vi "UIMessage AX Callback.vi"(4 "Variant":variant, 5 "Event Data":cluster{"msg":refnum<k7>}, 6 "Control Ref":refnum<k7>, 7 "Event Common Data":T2) -> ()   [LabVIEW 2020, in "TSnax.lvlib" / "Engine.lvclass"]
uses:
  Engine.lvclass
  UIMsg.ctl
  Engine.lvclass/Engine.ctl
  UIMessage/UIMessage.lvclass
  TSnax.lvlib
panel:
  out "Code":T1
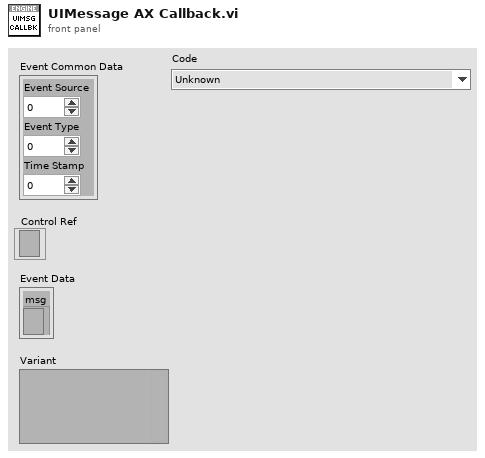
[diagram p1: front panel]
types:
  T1 = typedef "TSnax.lvlib/UIMsg.ctl" = enum16{"Unknown", "BreakOnUserRequest", "BreakOnBreakpoint", "BreakOnRunTimeError", "Trace", "TerminatingExecution", "AbortingExecution", "KillingExecutionThreads", "EndExecution", "ShutDownComplete", "StartExecution", "ProgressPercent", "ProgressText", "StartInteractiveExecution", "EndInteractiveExecution", "TerminatingInteractiveExecution", "TerminationCancelled", "ResumeFromBreak", "StartFileExecution", "EndFileExecution", "ShutDownCancelled", "LocalizationSettingChanged", "OpenWindows", "TileWindows", "CascadeWindows", "ReportChanged", "CloseWindows", "RefreshWindows", "ClientFileChanged", "DisplayReport", "ModelState_Initializing", "ModelState_Waiting", "ModelState_Identified", "ModelState_BeginTesting", "ModelState_TestingComplete", "ModelState_PostProcessingComplete", "ModelState_EnabledStateSet", "ReportLocationChanged", "GotoLocation", "PushUndoItem", "OutputMessages", "TypePaletteFileListChanged", "NonTerminatingThreadsArePreventingTermination", "ModelState_PostProcessing", "ReportCollectionChanged", "RuntimeError"}
  T2 = cluster{"Event Source":i32, "Event Type":u32, "Time Stamp":u32}
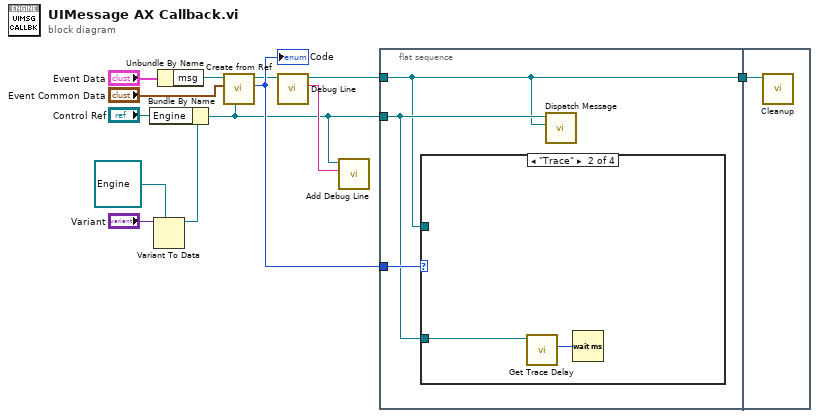
[diagram p0: block diagram]
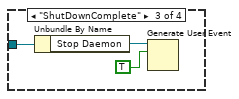
[diagram p3: hidden frame]
diagram:
  n1 = Variant To Data(type=refnum<class "Engine.lvclass"> refnum ("TSnax.lvlib:Engine.lvclass"), Variant="Variant") -> (data=w6:refnum<class "Engine.lvclass">)  [unwired: 1 in, 1 out]
  n2 = Bundle By Name(cluster=w6, "Engine"="Control Ref") -> (w1:refnum<class "Engine.lvclass">)
  n3 = Unbundle By Name("Event Data") -> ("msg"=w5:refnum<k7>)
  n4 = call "Create from Ref.vi"("TSnax:Engine"=w1, "Event Common Data"="Event Common Data", "msg"=w5) -> ("Code"=w4:T1, "UIMessage out"=w3:refnum<class "UIMessage.lvclass">)  [unwired: 6 in, 1 out]
  "Code" <- w4
  n5 = call "Debug Line.vi"("UIMessage in"=w3) -> ("Debug Line"=w8:string, "UIMessage out"=w10:refnum<class "UIMessage.lvclass">)  [unwired: 9 in]
  n6 = call "Add Debug Line.vi"("Debug Line"=w8, "Engine in"=w1) -> ()  [unwired: 10 in]
  n7 = flat-sequence {
    tunnel: w10 -> [w14]
    tunnel: [w14] -> w9
    tunnel: w1 -> [w15]
    tunnel: w4 -> [w16]
    tunnel: w9 -> [w22]
    frame #0 {
      n8 = case shown="\"Trace\"" w16 {
        tunnel: w14 -> [_ _ _ _]
        tunnel: w15 -> [_ w18 w21 _]
        frame Default {
        }
        frame "Trace" {
          n9 = call "Get Trace Delay.vi"("Engine in"=w18) -> ("Trace Delay ms"=w17:u32)  [unwired: 8 in, 2 out]
          n10 = Wait (ms)(milliseconds to wait=w17) -> ()  [unwired: 1 out]
        }
        frame "ShutDownComplete" {
          n11 = Unbundle By Name(w21) -> ("Stop Daemon"=w20:refnum<user-event>)
          n12 = Generate User Event(user event=w20, event data cluster=TRUE ("event data")) -> ()  [unwired: 2 in, 2 out]
        }
        frame "ShutDownCancelled" {
        }
      }
      n13 = call "Dispatch Message.vi"("TSnax:UIMessage"=w14, "Engine in"=w15) -> ()  [unwired: 8 in, 2 out]
    }
    frame #1 {
      n14 = call "Cleanup.vi"("UIMessage in"=w22) -> ()  [unwired: 10 in, 1 out]
    }
  }
